vi "BotSpeak_Set.vi"(2 "value":string, 3 "Variable In":string="power", 4 "Bot Settings":T1) -> (0 "response":string="169.254.32.85", 1 "Bot Settings":T1)   [LabVIEW 2012]
doc: "Sets the value of \"Variable in\" and returns that as \"value\"."
uses:
  <userlib>/BotSpeak/VIs/Direct/BotSpeak_Control.ctl
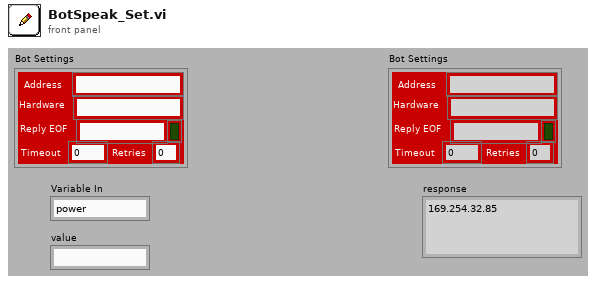
[diagram p1: front panel]
types:
  T1 = typedef "BotSpeak_Control.ctl" = cluster{"Address":string, "Reply EOF":string, "Hardware":string, "Retries":i8, "Timeout":i32, "Open?":bool}
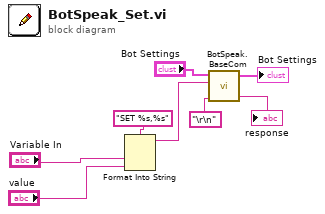
[diagram p0: block diagram]
diagram:
  n1 = Format Into String(format string="SET %s,%s" ("command"), "Variable In", "value") -> (resulting string=w8:string)  [unwired: 2 in, 1 out]
  n2 = call <userlib>:"BotSpeak.BaseCom.vi"("Termination"="\r\n", "command"=w8, "Bot Settings in"="Bot Settings") -> ("response"=→"response":string, "Bot Settings out"=→"Bot Settings":T1)  [unwired: 2 in]
